vi "Read DVR.vi"(8 "error in (no error)":errorcluster, 11 "Data DVR Session in":refnum<class "Data DVR Session.lvclass">) -> (0 "error out":errorcluster, 2 "DVR":refnum<data-value>, 3 "Data DVR Session out":refnum<class "Data DVR Session.lvclass">)   [LabVIEW 2014, in "Data DVR Session.lvclass"]
uses:
  Data DVR Session.lvclass
  Data/Data.lvclass
  Data DVR Session.lvclass/Data DVR Session.ctl
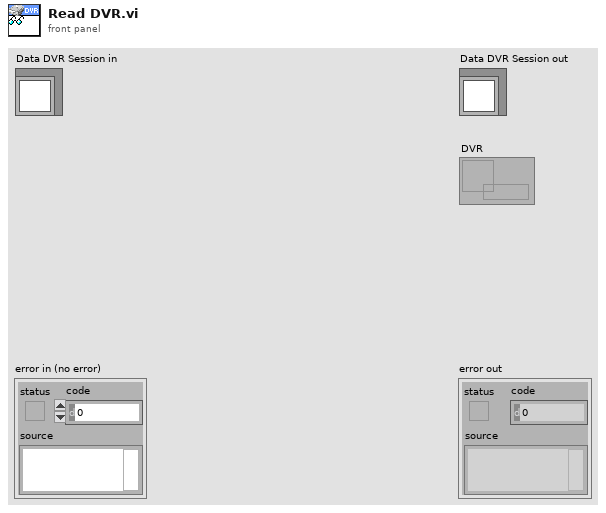
[diagram p1: front panel]
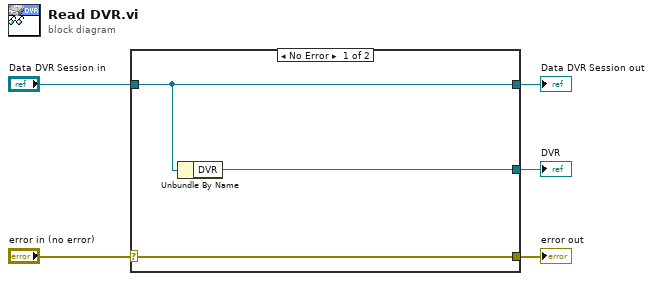
[diagram p0: block diagram]
diagram:
  n1 = case shown="No Error" "error in (no error)" {
    selector: "error in (no error)" -> [w8 w9]
    tunnel: [w8 w9] -> w4
    tunnel: [w7 w10] -> w2
    tunnel: "Data DVR Session in" -> [w7 w10]
    tunnel: [w6 _] -> w1
    frame No Error {
      n2 = Unbundle By Name(w7) -> ("DVR"=w6:refnum<data-value>)
    }
    frame Error {
    }
  }
  "error out" <- w4
  "Data DVR Session out" <- w2
  "DVR" <- w1
